vi "dispense test.vi"() -> ()   [LabVIEW 2019]
uses:
  Classes/Controller/Dispenser/Dispenser.lvclass
  Classes/Controller/Controller.lvclass
panel:
  in  "Stop":bool
  in  "Pressure":i16
  in  "Dispense":bool
  # "Make sure that Dispense is off before hitting stop. The Dispense command has to be sent to the Nordson box a second time to stop dispensing. Otherwise, dispensing will continue, even after this program is closed."
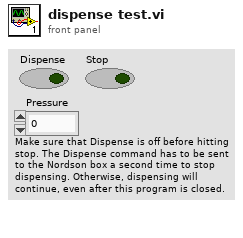
[diagram p1: front panel]
types:
  T1 = typedef "Controller.lvclass/Controllers.ctl" = cluster{"I-O.lvclass":refnum<class "I-O.lvclass">, "Dispenser.lvclass":refnum<class "Dispenser.lvclass">, "Gantry":refnum<k24>}
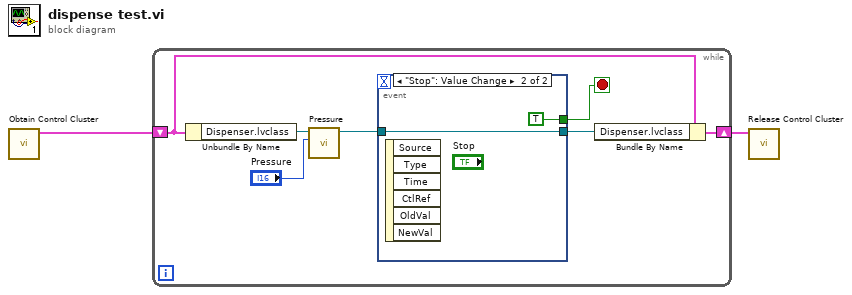
[diagram p0: block diagram]
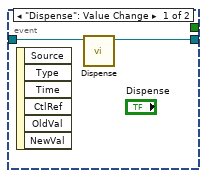
[diagram p2: hidden frame]
diagram:
  n1 = call "Obtain Control Cluster.vi"() -> ("Control Out"=w2:T1)  [unwired: 11 in]
  n2 = while {
    shift-right: [w4] -> w1
    shift-left: w2 -> [w6]
    stop <- w3 stop-if-true
    n3 = Unbundle By Name(w6) -> ("Dispenser.lvclass"=w9:refnum<class "Dispenser.lvclass">)
    n4 = call-dynamic "Pressure.vi"("Pressure"="Pressure", "Dispenser in"=w9) -> ("Dispenser out"=w7:refnum<class "Dispenser.lvclass">)  [unwired: 8 in, 1 out]
    n5 = event shown="[1] \"Stop\": Value Change" {
      selector: _ -> [_ _]
      dyn-events: _ -> [_ _]
      timeout: _ -> [_ _]
      tunnel: w7 -> [w11 w12]
      tunnel: [w10 w12] -> w5
      tunnel: [_ TRUE] -> w3
      event "Dispense": Value Change {
        n6 = event-data() -> ()  [unwired: 1 in, 6 out]
        n7 = call-dynamic "Dispense.vi"("Dispenser in"=w11) -> ("Dispenser out"=w10:refnum<class "Dispenser.lvclass">)  [unwired: 9 in, 1 out]
      }
      event "Stop": Value Change {
        n8 = event-data() -> ()  [unwired: 1 in, 6 out]
      }
    }
    n9 = Bundle By Name(cluster=w6, "Dispenser.lvclass"=w5) -> (w4:T1)
  }
  n10 = call "Release Control Cluster.vi"("output cluster"=w1) -> ()  [unwired: 11 in]
